vi "Extract row or column.vi"() -> ()   [LabVIEW 2012]
panel:
  in  "Option":string(combo)="Row"
  out "Array out":dbl[](array[numeric])=[2.1, 2.2, 2.3, 2.4]
  in  "Row/Column index":i32=1
  in  "Array":dbl[][](array[numeric])=[[1.1, 1.2, 1.3, 1.4], [2.1, 2.2, 2.3, 2.4], [3.1, 3.2, 3.2, 3.4], [4.1, 4.2, 4.3, 4.4], [5.1, 5.2, 5.3, 5.4]]
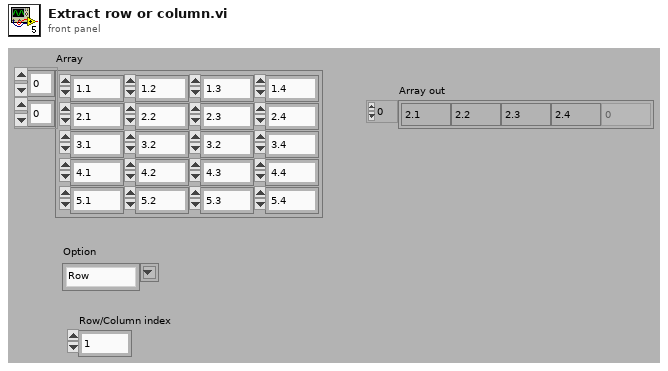
[diagram p1: front panel]
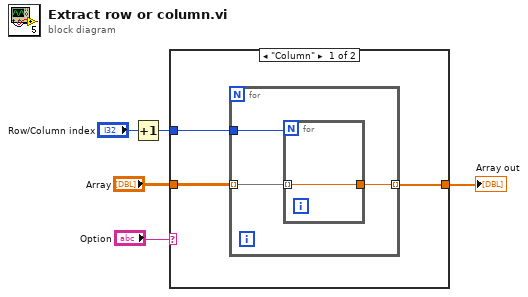
[diagram p0: block diagram]
diagram:
  n1 = Increment(x="Row/Column index") -> (x+1=w1:i32)
  n2 = case shown="\"Column\"" "Option" {
    tunnel: "Array" -> [w8 w15]
    tunnel: [w6 w14] -> w4
    tunnel: w1 -> [w7 w13]
    frame "Column" {
      n3 = for {
        tunnel: w8 -> [w10] mode=indexing
        tunnel: w7 -> [w11]
        tunnel: [w9] -> w6 mode=indexing
        n4 = for {
          N: w11 -> [_]
          tunnel: w10 -> [w12] mode=indexing
          tunnel: [w12] -> w9
        }
      }
    }
    frame "Row", Default {
      n5 = for {
        N: w13 -> [_]
        tunnel: w15 -> [w16] mode=indexing
        tunnel: [w16] -> w14
      }
    }
  }
  "Array out" <- w4
